vi "Calibration.vi"(4 "flush duration [s]":dbl, 7 "Desired Refresh Ratio":dbl=25.0 format="%#_g %", 8 "LINX Resource":T2={"IO"=enum."Remote", "Interface"=enum."TCP", "LINX Device Config"={"Interface"=enum."Serial", "COM Port"="COM13", "TCP Configuration"={"IP Address"="", "Port"=0}, "Device Family"=1, "Device ID"=1, "Device Name"="myRIO-1900", "TCP Ref"=refnum, "Channels"={"DI"=[0, 1, 2, 3, 4, 5, 6, 7, 8, 9, 10, 11, 12, 13, 14, 15, 16, 17, 18, 19, 20, 21, 22, 23, 24, 25, 26, 27, 28, 29, 30, 31, 32, 33, 34, 35, 36, 37, 38, 39, 40, 41, 42, 43, 44, 45, 46], "DO"=[0, 1, 2, 3, 4, 5, 6, 7, 8, 9, 10, 11, 12, 13, 14, 15, 16, 17, 18, 19, 20, 21, 22, 23, 24, 25, 26, 27, 28, 29, 30, 31, 32, 33, 34, 35, 36, 37, 38, 39, 40, 41, 42, 43, 44, 45, 46], "AI"=[0, 1, 2, 3, 4, 5, 6, 7, 8, 9, 10, 11], "AO"=[], "PWM"=[3, 5, 6, 9, 10], "QE"=[], "UART"=[0, 1], "I2C 2"=[0], "SPI"=[0], "CAN"=[], "Servo"=[], "AI Ref (V)"=0.0, "AI Resolution (Bits)"=0, "AO Ref (V)"=0.0, "AO Resolution (Bits)"=0}}}, 9 "SOLA ID":u32, 10 "TANGO ID":i32, 11 "IX 81 Port":refnum<visa-resource-name>="IX2-UCB") -> (0 "error IO":errorcluster, 2 "CalibFile":path, 3 "Number of pump steps\n for the desired refresh ratio":dbl)   [LabVIEW 2018]
doc: "This template is for the Queued Message Handler design pattern.\n\nThe Event Handling Loop generates messages based on user interface actions.\n\nThe Message Handling Loop processes messages generated by the Event Handling Loop, or by other messages. The messages are string values, so new messages can be added easily to the Message Cases case structure in the Message Handling Loop. Each message cluster can also provide an optional value for Message Data, which is a variant that can be converted to whatever message-specific data is required."
uses:
  ANDOR/OwnVIs/AndorOWN.lvlib
  SOLA/LabVIEW 2015 Library (32bit)/LumencorDLL32/LumencorDLL32.lvlib
  Olympus IX BX Series/Olympus IX BX Series.lvlib
  TANGO Stage/TangoOWN.lvlib
  <vilib>/MakerHub/LINX/LMH-LINX.lvlib
  Arduino/VIs/Arduino.lvlib
  ANDOR/Andor SDK/AndorSDK.lvlib
  <vilib>/vision/NI_Vision_Development_Module.lvlib
  tiff/LVTiffWriter/LVTiffWriter.lvlib
  <vilib>/MakerHub/LINX/Public/Peripherals/Digital/Digital Write N Chans.vi
  Calib/Calibration.lvlib
  <vilib>/MakerHub/LINX/Private/Type Defs/Platform.ctl
  <vilib>/MakerHub/LINX/Private/Type Defs/Interface.ctl
  <vilib>/MakerHub/LINX/Private/Device/Type Defs/TCP Config.ctl
  <vilib>/MakerHub/LINX/Private/Device/Device.lvlib
  <vilib>/MakerHub/LINX/Private/Device/Type Defs/Channels.ctl
  <vilib>/MakerHub/LINX/Private/Device/Type Defs/LINX Device Config.ctl
  <vilib>/MakerHub/LINX/Private/Type Defs/LINX Ref.ctl
  C:/Users/Familie/Documents/LabviewIX81/lib/tiff/LVTiffWriter/BitMiracle.LibTiff.NET.dll
  tiff/LVTiffWriter/BitMiracle.LibTiff.NET.dll
panel:
  out "function return":u32
  out "color":string
  in  "Messages":string
  out "TiffHandle":refnum<k24>
  in  "Image Name":string="TestIMG"
  out "Acq. Error Array":cluster{i32, string}[](array[cluster])
  in  "Single Image":bool
  out "Image":T1(plugin-control)
  in  "Colormap":u16(ring) items=["Grey", "Hot"]
  in  "Format":u16(ring)=6
  in  "Path":path
  in  "Save Image":bool
  in  "Exposure 2":sgl=50.0 format="%#_g ms"
  in  "Filter":u16(ring) items=["UV ", "CFP", "GFP", "YFP", "RFP", "BF (empty)"]
  out "exposure out":sgl
  out "accumulate out":sgl
  out "kinetic out":sgl
  out "Camera Temperature":sgl format="%.2f °C"
  in  "Calibrate at Startup":bool
  out "Y Limits":dbl[](array[numeric]) caption="Y Limits [µm]" format="%#_12f"
  out "X Limits":dbl[](array[numeric]) caption="X Limits [µm]" format="%#_10f"
  out "Lower Limit":dbl
  out "Upper Limit":dbl
  in  "Focus [um]":dbl format="%.3f"
  in  "Intensity [%]":dbl(slide) scale=0.0..100.0 scale format="%.1f"
  in  "Light Source":u16(ring) items=["BF - Lamp", "SOLA"]
  in  "Prism Position (1: Bi)":enum16{"Bi", "Side"}(ring)=enum."Side"
  in  "Objective":enum16{"x 4", "x 10", "x 20", "x 40", "x 100"}(ring)=enum."x 10"
  in  "Lamp Type (0: Transmitted)":enum16{"Transmitted", "Reflected"}(ring)
  in  "Enable Lamp":bool
  in  "Shutter":bool
  in  "Microscope Settings":i32(listbox)
  out "Slide":u8(slide) scale=0.0..100.0
  in  "Valve Actuation":i32(listbox)
  in  "Configuration File Path":path
  in  "stop":bool
  out "error out":errorcluster
  in  "Position List":i32[](listbox)
  out "Tango Success":bool
  in  "TANGO COM Port":refnum<visa-resource-name>="COM4"
  in  "SOLA COM Port":refnum<visa-resource-name>="COM5"
  in  "Valve Port (Arduino)":refnum<visa-resource-name>="COM7"
  # "Initialization"
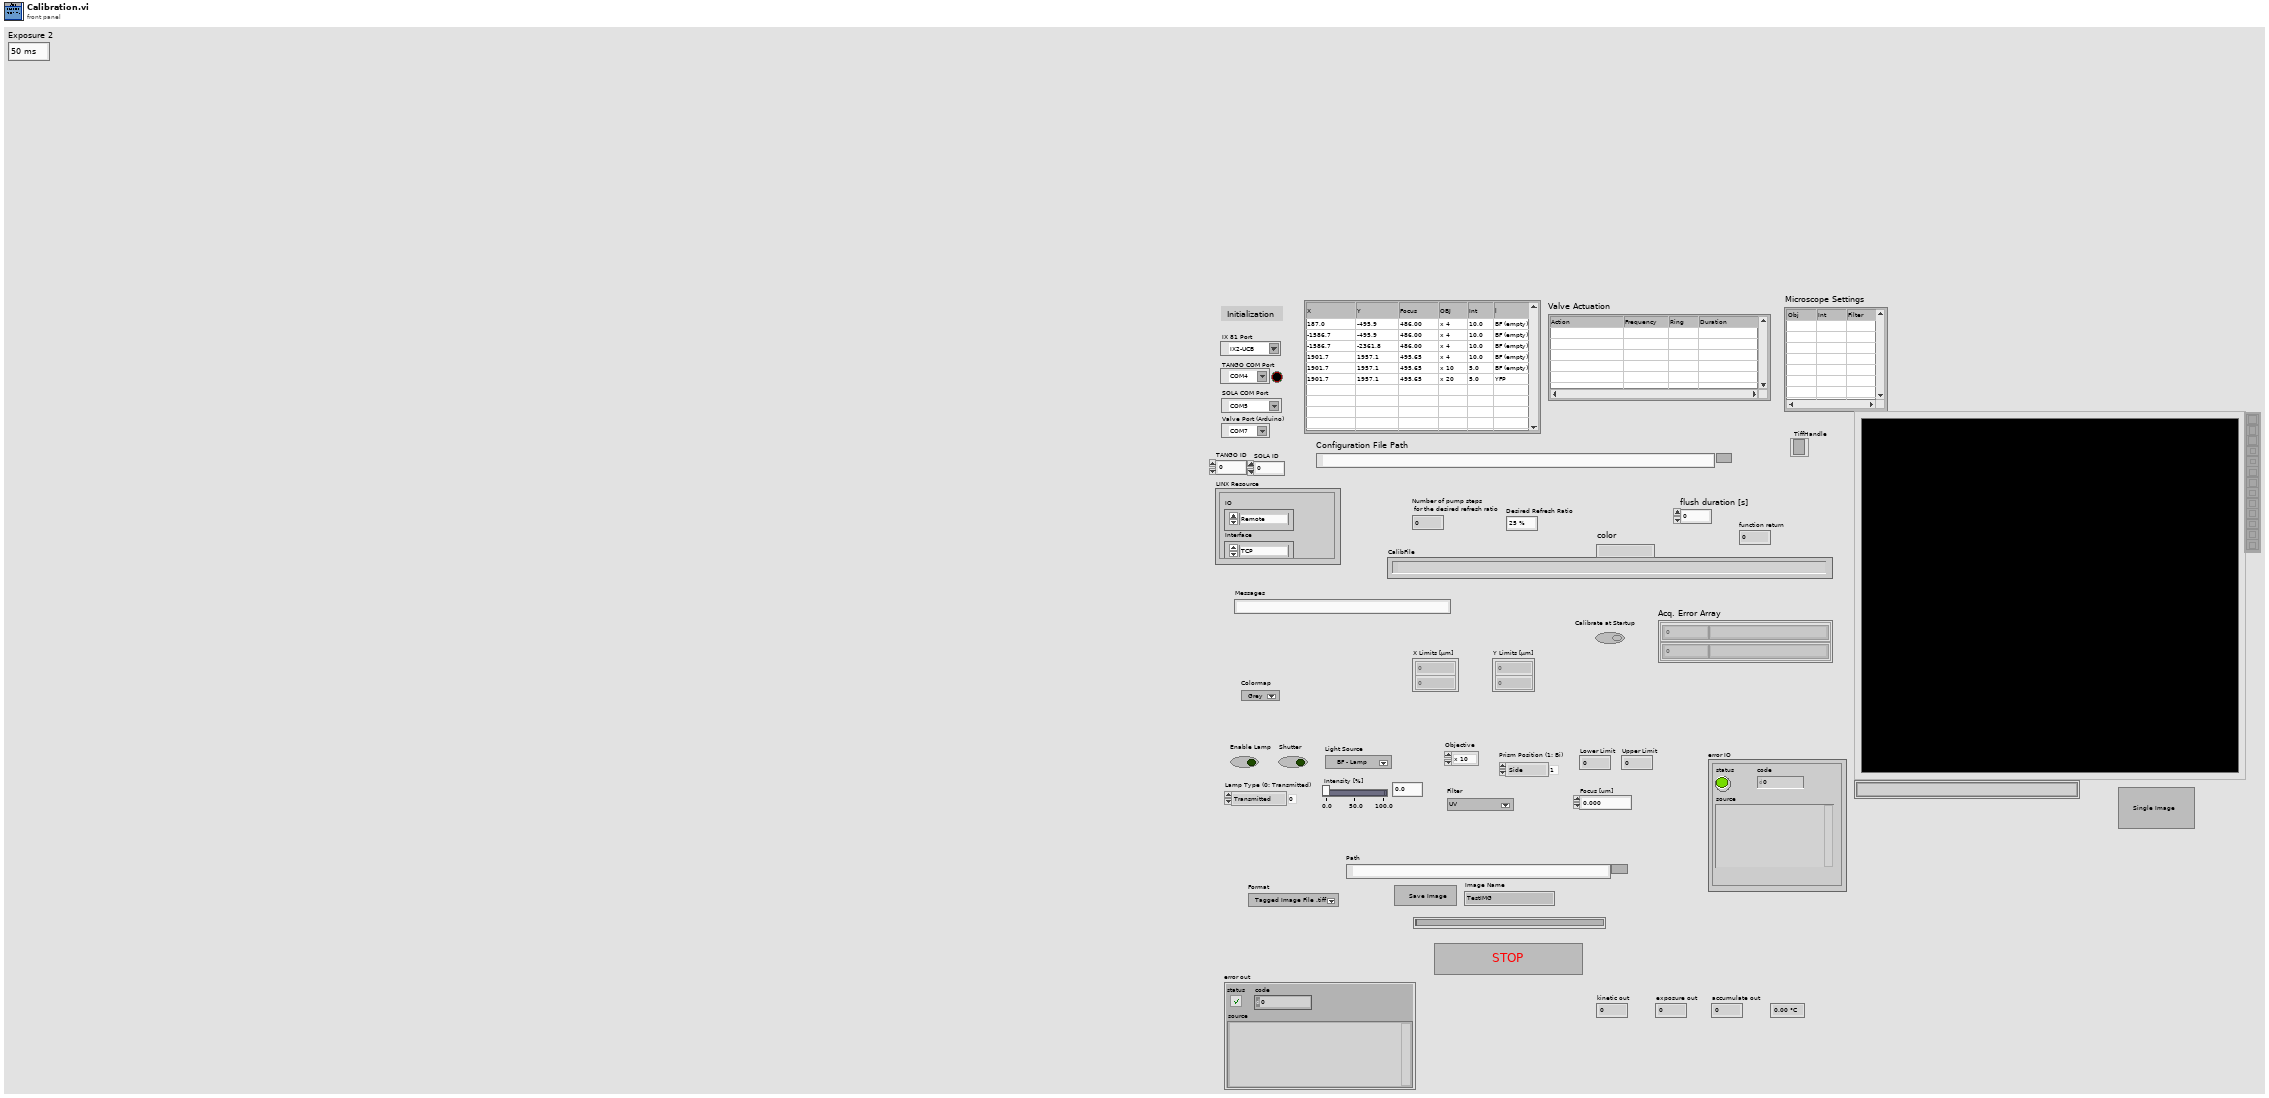
[diagram p1: front panel]
types:
  T1 = typedef "IMAQ Image.ctl" = refnum<image>
  T2 = typedef "LMH-LINX.lvlib/LINX Ref.ctl" = cluster{"IO":T3, "Interface":T4, "LINX Device Config":T5}
  T3 = typedef "LMH-LINX.lvlib/Platform.ctl" = enum16{"Remote", "Local"}
  T4 = typedef "LMH-LINX.lvlib/Interface.ctl" = enum16{"Serial", "TCP"}
  T5 = typedef "LMH-LINX.lvlib/Device.lvlib/LINX Device Config.ctl" = cluster{"Interface":T4, "COM Port":refnum<visa-resource-name>, "TCP Configuration":T6, "Device Family":u8, "Device ID":u8, "Device Name":string, "TCP Ref":refnum<k5>, "Channels":T7}
  T6 = typedef "LMH-LINX.lvlib/Device.lvlib/TCP Config.ctl" = cluster{"IP Address":string, "Port":u16}
  T7 = typedef "LMH-LINX.lvlib/Channels.ctl" = cluster{"DI":u8[], "DO":u8[], "AI":u8[], "AO":u8[], "PWM":u8[], "QE":u8[], "UART":u8[], "I2C 2":u8[], "SPI":u8[], "CAN":u8[], "Servo":u8[], "AI Ref (V)":dbl, "AI Resolution (Bits)":u8, "AO Ref (V)":dbl, "AO Resolution (Bits)":u8}
  T8 = enum16{"open", "replace", "create", "open or create", "replace or create", "replace or create with confirmation"}
  T9 = typedef "Image Type" = u32
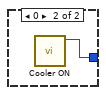
[diagram p2: hidden frame]
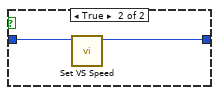
[diagram p3: hidden frame]
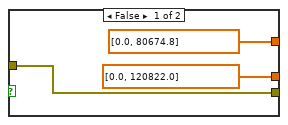
[diagram p4: hidden frame]
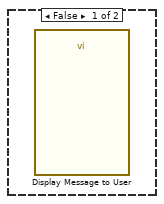
[diagram p6: hidden frame]
diagram:
  n1 = flat-sequence {
    tunnel: [errorcluster {"status"=FALSE, "code"=0, "source"=""} ("error IO")] -> w2
    tunnel: w2 -> [w5]
    tunnel: [w4] -> w1
    tunnel: w1 -> [_]
    frame #0 {
    }
    frame #1 {
      w67 = 0  # openingtime
      w65 = 0  # Auto Mode
      w64 = 1  # TTL High to open
      w66 = 0  # closingtime
      w63 = 0  # Internal Trigger
      w61 = 1  # Single Scan
      w62 = 4  # Image Read
      n2 = call "Is Cooler On.vi"() -> ("function return"=w50:u32, "iCoolerStatus out"=w51:i32)  [unwired: 9 in, 1 out]
      n3 = local read "Calibrate at Startup"() -> (w84:bool)
      n4 = call "lm Color Level.vi"("error in (no error)"=w5, "str_Level"="100", "str_Color"="WHITE") -> ("error out"=w86:errorcluster, "str_Color out"=w87:string)  [unwired: 6 in, 1 out]
      n5 = call "Get VS Speed.vi"() -> ("speed out"=w70:sgl, "function return"=w37:u32)  [unwired: 9 in, 1 out]
      n6 = call "Get Fastest Recommended VS Speed.vi"() -> ("function return"=w36:u32, "speed out"=w69:sgl, "index out"=w72:i32)  [unwired: 8 in, 1 out]
      n7 = case shown="1, Default" w51 {
        tunnel: [u32 20002 ("function return") w91] -> w49
        frame 1, Default {
        }
        frame 0 {
          n8 = call "Cooler ON.vi"() -> ("function return"=w91:u32)  [unwired: 10 in, 1 out]
        }
      }
      n9 = Greater Or Equal?(x=w69, y=w70) -> (x >= y?=w71:bool)
      n10 = call "AndorCreaterErrorCluster.vi"() -> ("Error Code Array"=w35:cluster{i32, string}[])  [unwired: 11 in]
      n11 = call "lm Color Enable.vi"("error in (no error)"=w86, "str_State"="ON", "str_Color"=w87) -> ("error out"=w75:errorcluster)  [unwired: 6 in, 2 out]
      n12 = case shown="True" w84 {
        tunnel: [w95 w102] -> w74
        tunnel: w5 -> [w95 w98]
        tunnel: [dbl[] [0.0, 80674.8] ("Y Limits") w101] -> w82
        tunnel: [dbl[] [0.0, 120822.0] ("X Limits") w100] -> w83
        frame False {
        }
        frame True {
          n13 = local read "TANGO ID"() -> (w99:i32)
          n14 = call "TangoCalibrate.vi"("error in (no error)"=w98, "plLSID in"=w99) -> ("error out"=w102:errorcluster, "X Limits"=w100:dbl[], "Y Limits"=w101:dbl[])  [unwired: 7 in]
        }
      }
      n15 = case shown="False" w71 {
        tunnel: w72 -> [_ w94]
        tunnel: [u32 20002 ("function return") w93] -> w38
        frame False {
        }
        frame True {
          n16 = call "Set VS Speed.vi"("index"=w94) -> ("function return"=w93:u32)  [unwired: 10 in]
        }
      }
      n17 = call "AndorReturn2Error.vi"(9:w35, "Camera return"=w50) -> ("error out"=w33:errorcluster, 3:w34)  [unwired: 8 in]
      n18 = call "AndorReturn2Error.vi"("error in (no error)"=w33, 9:w34, "Camera return"=w49) -> ("error out"=w32:errorcluster, 3:w6)  [unwired: 7 in]
      n19 = call "AndorReturn2Error.vi"("error in (no error)"=w32, 9:w6, "Camera return"=w36) -> ("error out"=w31:errorcluster, 3:w7)  [unwired: 7 in]
      n20 = call "AndorReturn2Error.vi"("error in (no error)"=w31, 9:w7, "Camera return"=w37) -> ("error out"=w30:errorcluster, 3:w8)  [unwired: 7 in]
      n21 = call "AndorReturn2Error.vi"("error in (no error)"=w30, 9:w8, "Camera return"=w38) -> ("error out"=w29:errorcluster, 3:w9)  [unwired: 7 in]
      n22 = call "Get Temperature F.vi"() -> ("function return"=w39:u32, "temperature out"=w68:sgl)  [unwired: 9 in, 1 out]
      n23 = local read "LINX Resource"() -> (w81:T2)
      n24 = local write "Y Limits"(w82) -> ()
      n25 = local write "X Limits"(w83) -> ()
      n26 = local write "Camera Temperature"(w68) -> ()
      n27 = call "AndorReturn2Error.vi"("error in (no error)"=w29, 9:w9, "Camera return"=w39) -> ("error out"=w28:errorcluster, 3:w10)  [unwired: 7 in]
      n28 = call "Set Read Mode.vi"("mode"=w62) -> ("function return"=w40:u32)  [unwired: 9 in, 1 out]
      n29 = call "ArdnoValve2Linx.vi"("error in (no error)"=w5, "Valve (A1-C8),\n comma separated"="A1,A2,A3,A4,A5,A6,A7,A8,B1,B2,B3,B4,B5,B6,B7,B8,C1,C2,C3,C4,C5,C6,C7,C8" ("Valve (A1-C8),\n comma separated")) -> ("error out"=w79:errorcluster, "Closed State"=w78:bool[], "Linx Port"=w77:i32[])  [unwired: 7 in]
      n30 = call "Set Shutter.vi"("openingtime"=w67, "closingtime"=w66, "mode"=w65, "typ"=w64) -> ("function return"=w41:u32)  [unwired: 6 in, 1 out]
      n31 = call "AndorReturn2Error.vi"("error in (no error)"=w28, 9:w10, "Camera return"=w40) -> ("error out"=w27:errorcluster, 3:w11)  [unwired: 7 in]
      n32 = call-poly <vilib>:"Digital Write.vi"("Error In"=w79, "Values"=w78, "DO Channels"=w77, "LINX Resource"=w81) -> ("Error Out"=w76:errorcluster)  [unwired: 6 in, 1 out]
      n33 = call "AndorReturn2Error.vi"("error in (no error)"=w27, 9:w11, "Camera return"=w41) -> ("error out"=w26:errorcluster, 3:w12)  [unwired: 7 in]
      n34 = call "Set Trigger Mode.vi"("mode"=w63) -> ("function return"=w42:u32)  [unwired: 9 in, 1 out]
      n35 = call "Set Acquisition Mode.vi"("mode"=w61) -> ("function return"=w43:u32)  [unwired: 9 in, 1 out]
      n36 = call "AndorReturn2Error.vi"("error in (no error)"=w26, 9:w12, "Camera return"=w42) -> ("error out"=w25:errorcluster, 3:w13)  [unwired: 7 in]
      n37 = call "AndorReturn2Error.vi"("error in (no error)"=w25, 9:w13, "Camera return"=w43) -> ("error out"=w24:errorcluster, 3:w14)  [unwired: 7 in]
      n38 = call "Set Temperature.vi"("temperature"=-60) -> ()  [unwired: 9 in, 2 out]
      n39 = call "Set Frame Transfer Mode.vi"("mode"=1) -> ("function return"=w44:u32)  [unwired: 10 in]
      n40 = call "AndorReturn2Error.vi"("error in (no error)"=w24, 9:w14, "Camera return"=w44) -> ("error out"=w23:errorcluster, 3:w15)  [unwired: 7 in]
      n41 = local read item#-1() -> (w57)
      n42 = call "Set Number Accumulations.vi"("number"=1) -> ("function return"=w45:u32)  [unwired: 9 in, 1 out]
      n43 = call "AndorReturn2Error.vi"("error in (no error)"=w23, 9:w15, "Camera return"=w45) -> ("error out"=w22:errorcluster, 3:w16)  [unwired: 7 in]
      n44 = Divide(x=w57, y=sgl 1000.0) -> (x/y=w56:sgl)
      n45 = call "Set Number Kinetics.vi"("number"=1) -> ("function return"=w46:u32)  [unwired: 9 in, 1 out]
      n46 = call "Set Exposure Time.vi"("time"=w56) -> ("function return"=w47:u32)  [unwired: 9 in, 1 out]
      n47 = call "AndorReturn2Error.vi"("error in (no error)"=w22, 9:w16, "Camera return"=w46) -> ("error out"=w21:errorcluster, 3:w17)  [unwired: 7 in]
      n48 = call "AndorReturn2Error.vi"("error in (no error)"=w21, 9:w17, "Camera return"=w47) -> ("error out"=w20:errorcluster, 3:w18)  [unwired: 7 in]
      n49 = call "Get Acquisition Timings.vi"() -> ("kinetic out"=w54:sgl, "accumulate out"=w52:sgl, "exposure out"=w53:sgl, "function return"=w48:u32)  [unwired: 7 in, 1 out]
      n50 = call "AndorReturn2Error.vi"("error in (no error)"=w20, 9:w18, "Camera return"=w48) -> ("error out"=w19:errorcluster)  [unwired: 8 in]
      n51 = local write "exposure out"(w53) -> ()
      n52 = local write "accumulate out"(w52) -> ()
      n53 = local write "kinetic out"(w54) -> ()
      n54 = Merge Errors(w76, w75, w74, w19) -> (w4:errorcluster)
    }
    frame #2 {
      n55 = Two Button Dialog(message="Do you want to calibrate the pumps now?") -> (T button?=w103:bool)  [unwired: 2 in]
      n56 = case shown="True" w103 {
        frame False {
        }
        frame True {
          n57 = flat-sequence {
            tunnel: [w149] -> w107
            tunnel: w107 -> [w153]
            tunnel: [w153] -> w106
            tunnel: [w151] -> w105
            tunnel: w106 -> [w155]
            tunnel: w105 -> [w154]
            frame #0 {
              n58 = Open/Create/Replace File(prompt="Specify the .tif file to save the images in.", operation (0:open)=T8."create", access (0:read/write)=enum16{"read/write", "read-only", "write-only"}."read/write") -> (refnum out=w111:refnum<file>, error out=w112:errorcluster)  [unwired: 3 in, 1 out]
              n59 = Close File(refnum=w111, error in=w112) -> (path=w110:path)  [unwired: 1 out]
              "CalibFile" <- w110
              n60 = call "tiffOpenForWrite.vi"("Path"=w110) -> ("TiffOut"=→"TiffHandle":refnum<k24>)  [unwired: 10 in]
            }
            frame #1 {
              w121 = u16 1 items=["BF - Lamp", "SOLA"] ("Light Source")
              n61 = call "Exposure Time check"() -> ("Color"=w115:string, "Exposure Time  [ms]"=w116:dbl)  [unwired: 16 in, 2 out]
              "color" <- w115
              n62 = local write "Light Source"(w121) -> ()
              n63 = property on="Filter" class="Ring (strict)"() -> ("Strings []"=w120:string[])  [unwired: 2 in, 2 out]
              n64 = Array Size(array=w120) -> (size(s)=w118:i32)
              n65 = flat-sequence {
                tunnel: [w134] -> w122
                tunnel: w116 -> [w135]
                tunnel: w122 -> [w145]
                frame #0 {
                  n66 = while {
                    tunnel: w135 -> [w136]
                    tunnel: [w136] -> w134
                    stop <- w137 stop-if-true
                    n67 = call "Get Status.vi"() -> ("function return"=w143:u32, "status out"=w140:i32)  [unwired: 9 in, 1 out]
                    n68 = Equal?(x=20073 ("status out"), y=w140) -> (x = y?=w139:bool)
                    n69 = Equal?(x=w143, y=20002 ("x")) -> (x = y?=w138:bool)
                    n70 = And(x=w139, y=w138) -> (x .and. y?=w137:bool)
                  }
                }
                frame #1 {
                  n71 = Divide(x=w145, y=sgl 1000.0) -> (x/y=w147:dbl)
                  n72 = call "Set Exposure Time.vi"("time"=w147) -> ("function return"=→"function return":u32)  [unwired: 9 in, 1 out]
                }
              }
              n73 = for {
                N: w118 -> [_]
                tunnel: w120 -> [w132] mode=indexing
                tunnel: w115 -> [w131]
                tunnel: [w130] -> w117
                i -> [w130]
                stop <- w133 stop-if-true
                n74 = Equal?(x=w131, y=w132) -> (x = y?=w133:bool)
              }
              n75 = local write item#-1(w116) -> ()
              n76 = Less?(x=w117, y=w118) -> (x < y?=w119:bool)
              n77 = case shown="True" w119 {
                tunnel: w117 -> [_ w126]
                frame False {
                  n78 = call "Display Message to User"() -> ()  [unwired: 10 in, 2 out]
                }
                frame True {
                  n79 = Increment(x=w126) -> (x+1=w125:i32)
                  n80 = Number To Decimal String(number=w125) -> (decimal integer string=w127:string)  [unwired: 1 in]
                  n81 = call <vilib>:"Space Constant.vi"() -> ("String"=w129:string)
                  n82 = local read "IX 81 Port"() -> (w123:refnum<visa-resource-name>)
                  n83 = Concatenate Strings("MU", w129, w127) -> (w124:string)
                  n84 = call "OlympusQuery.vi"("String"=w124, "VISA Resource Name In"=w123) -> ()  [unwired: 7 in, 3 out]
                }
              }
            }
            frame #2 {
            }
            frame #3 {
              n85 = local read "LINX Resource"() -> (w150:T2)
              n86 = One Button Dialog(message="Please load the fluorophore now") -> ()  [unwired: 1 in, 1 out]
              n87 = call "AndorConvertErrCodeToMessage.vi"(11:w150) -> (3:w149)  [unwired: 9 in, 1 out]
            }
            frame #4 {
              n88 = One Button Dialog(message="Please load the dilutant now") -> (true=w151:bool)  [unwired: 1 in]
            }
            frame #5 {
              n89 = case shown="True" w154 {
                tunnel: w155 -> [_ w156]
                frame False {
                }
                frame True {
                  n90 = flat-sequence {
                    tunnel: [w161] -> w159
                    tunnel: w156 -> [w160]
                    tunnel: w159 -> [w166]
                    tunnel: [w166] -> w158
                    tunnel: w158 -> [w169]
                    tunnel: [w167] -> w157
                    frame #0 {
                      n91 = call "ArdnoFlush.vi"("Open?"=FALSE, "Single / Multivalve?"=FALSE, "Channel"=u32 1, "LINX Resource"=w160) -> ("LINX Resource out"=w161:T2)  [unwired: 6 in, 1 out]
                    }
                    frame #1 {
                      n92 = Wait (ms)(milliseconds to wait="flush duration [s]") -> ()  [unwired: 1 out]
                    }
                    frame #2 {
                      (unwired) u32 1 ("Channel")
                      n93 = call "ArdnoFlush.vi"("Open?"=TRUE, "Single / Multivalve?"=FALSE, "LINX Resource"=w169) -> ("LINX Resource out"=w167:T2)  [unwired: 7 in, 1 out]
                    }
                  }
                  n94 = while {
                    tunnel: w157 -> [w178]
                    i -> [w175]
                    stop <- w172 continue-if-true
                    n95 = flat-sequence {
                      tunnel: w178 -> [w186]
                      tunnel: [w182] -> w177
                      tunnel: [w181] -> w176
                      tunnel: w177 -> [w191]
                      tunnel: w176 -> [w190]
                      tunnel: w175 -> [w192]
                      frame #0 {
                        w180 = u32 8  # Frequency
                        w184 = 15  # Feed Cycles
                        w185 = u32 1  # Channel
                        n96 = call "ArdnoFeed.vi"("LINX Resource"=w186, "Single / Multiring?"=FALSE ("Single / Multivalve?"), "Channel"=w185, "Feed Cycles"=w184, 13:w180) -> ("LINX Resource out"=w182:T2, "error out"=w181:errorcluster)  [unwired: 8 in, 1 out]
                      }
                      frame #1 {
                        w187 = 10  # Pump Frequency
                        w189 = 4  # Pump Cycles
                        n97 = call "ArdnoPump.vi"("LINX Resource"=w191, "Pump Cycles"=w189, "Pump Frequency"=w187, "error in (no error)"=w190, "Single/\nMultiring?"=FALSE ("Single/\nMultiring?")) -> ()  [unwired: 2 out]
                      }
                      frame #2 {
                        n98 = flat-sequence {
                          tunnel: TRUE ("NewVal") -> [w201]
                          tunnel: [w201] -> w196
                          tunnel: [w205] -> w195
                          tunnel: w196 -> [w205]
                          tunnel: w193 -> [w207]
                          tunnel: w195 -> [w208]
                          tunnel: w192 -> [w206]
                          frame #0 {
                            w199 = 1  # Single Scan
                            w200 = 4  # Image Read
                            n99 = call "Set Number Accumulations.vi"("number"=1) -> ()  [unwired: 9 in, 2 out]
                            n100 = call "Set Acquisition Mode.vi"("mode"=w199) -> ()  [unwired: 9 in, 2 out]
                            n101 = call "Set Read Mode.vi"("mode"=w200) -> ()  [unwired: 9 in, 2 out]
                            n102 = call "Set Number Kinetics.vi"("number"=1) -> ()  [unwired: 9 in, 2 out]
                          }
                          frame #1 {
                            n103 = local read item#-1() -> (w202)
                            n104 = Divide(x=w202, y=sgl 1000.0) -> (x/y=w204:sgl)
                            n105 = call "Set Exposure Time.vi"("time"=w204) -> ()  [unwired: 9 in, 2 out]
                          }
                          frame #2 {
                            n106 = case shown="True" w208 {
                              tunnel: w207 -> [_ w219]
                              tunnel: w206 -> [_ w209]
                              frame False {
                              }
                              frame True {
                                n107 = flat-sequence {
                                tunnel: w219 -> [w220]
                                tunnel: [w222] -> w218
                                tunnel: [w221] -> w217
                                tunnel: w218 -> [w224]
                                tunnel: w217 -> [w225]
                                tunnel: [w225] -> w216
                                tunnel: [w224] -> w215
                                tunnel: w216 -> [w240]
                                tunnel: w215 -> [w239]
                                tunnel: [w240] -> w214
                                tunnel: [w239] -> w213
                                tunnel: [w235] -> w212
                                tunnel: [w236] -> w211
                                tunnel: w214 -> [w244]
                                tunnel: w213 -> [w242]
                                tunnel: w212 -> [w243]
                                tunnel: w211 -> [w246]
                                tunnel: [w246] -> w210
                                tunnel: w210 -> [w269]
                                tunnel: w209 -> [w249]
                                frame #0 {
                                n108 = call "Start Acquisition.vi"() -> ("function return"=w223:u32)  [unwired: 10 in, 1 out]
                                n109 = call "Calibration.vi"("LINX Resource"=w223, "IX 81 Port"=w220) -> ("error IO"=w221:errorcluster, "Number of pump steps\n for the desired refresh ratio"=w222:dbl)  [unwired: 7 in, 1 out]
                                }
                                frame #1 {
                                n110 = while {
                                stop <- w226 stop-if-true
                                n111 = call "Get Status.vi"() -> ("function return"=w232:u32, "status out"=w229:i32)  [unwired: 9 in, 1 out]
                                n112 = Equal?(x=20073 ("status out"), y=w229) -> (x = y?=w228:bool)
                                n113 = Equal?(x=w232, y=20002 ("x")) -> (x = y?=w227:bool)
                                n114 = And(x=w228, y=w227) -> (x .and. y?=w226:bool)
                                }
                                }
                                frame #2 {
                                n115 = Square(x=1024) -> (x^2=w233:i32)
                                n116 = Initialize Array(i16 0 ("element"), w233) -> (w234:i16[])
                                n117 = call "Get Most Recent Image16.vi"("size"=w233, "arr"=w234) -> ("function return"=w235:u32, "arr out"=w236:i16[])  [unwired: 7 in, 1 out]
                                }
                                frame #3 {
                                n118 = call "Calibration.vi"("LINX Resource"=w243, "IX 81 Port"=w242) -> ("error IO"=w245:errorcluster)  [unwired: 7 in, 2 out]
                                n119 = Build Array(w245, w244) -> (w241:errorcluster[])
                                n120 = local write "Acq. Error Array"(w241) -> ()
                                }
                                frame #4 {
                                w272 = u32 2 items=["Zero Order", "Bi-Linear", "Quadratic", "Cubic Spline"] ("Interpolation Type")
                                w271 = T9 7 items=["Grayscale (U8)", "Grayscale (I16)", "Grayscale (SGL)", "Complex (CSG)", "RGB (U32)", "HSL (U32)", "RGB (U64)", "Grayscale (U16)"] ("Image Type")
                                w270 = 1024 ("dimension size")
                                n121 = Add(x=1 ("y"), y=w249) -> (x+y=w254:i32)
                                n122 = local read "Image Name"() -> (w268:string)
                                n123 = Reshape Array(w269, w270, w270) -> (w248:i16[][])
                                n124 = To Unsigned Word Integer(number=w248) -> (unsigned 16bit integer=w247:u16[][])
                                n125 = call "IMAQ Create"("Image Name"=w268, "Image Type"=w271) -> ("New Image"=w273:T1)  [unwired: 3 in, 1 out]
                                n126 = Bundle By Name(cluster=cluster{"Page":i32, "TotalPages":i32} {"Page"=0, "TotalPages"=0} ("Multipage"), "TotalPages"=10, "Page"=w254) -> (w256:cluster{"Page":i32, "TotalPages":i32})
                                n127 = local read "TiffHandle"() -> (w258:refnum<k24>)
                                n128 = call "IMAQ ArrayToImage"("Image Pixels (U16)"=w247, "Image"=w273) -> ("Image Out"=w253:T1)  [unwired: 8 in, 1 out]
                                n129 = property on="Image" class="ImageControl"() -> ("Image Area Height"=w266:u32, "Image Area Width"=w267:u32)  [unwired: 2 in, 2 out]
                                n130 = call "tiffWriteImaqToTiff.vi"("Multipage"=w256, "ImaqIn"=w253, "TiffIn"=w258) -> ("ImaqOut"=w252:T1, "TiffOut"=w259:refnum<k24>)  [unwired: 7 in]
                                n131 = call "IMAQ GetImageSize"("Image"=w253) -> ("Y Resolution"=w260:i32, "X Resolution"=w263:i32)  [unwired: 3 in, 1 out]
                                n132 = Divide(x=w260, y=w266) -> (x/y=w274:dbl)
                                n133 = Divide(x=w263, y=w267) -> (x/y=w275:dbl)
                                n134 = local write "TiffHandle"(w259) -> ()
                                n135 = Max & Min(x=w274, y=w275) -> (max(x,y)=w265:dbl, min(x,y)=w261:dbl)
                                n136 = Divide(x=w263, y=w265) -> (x/y=w264:dbl)
                                n137 = Divide(x=w260, y=w261) -> (x/y=w262:dbl)
                                n138 = call "IMAQ Resample"("X Resolution"=w264, "Y Resolution"=w262, "Interpolation Type"=w272, "Image Src"=w252) -> ("Image Dst Out"=w251:T1)  [unwired: 6 in, 1 out]
                                n139 = local write "Image"(w251) -> ()
                                }
                                }
                              }
                            }
                          }
                        }
                        n140 = call "AndorCreaterErrorCluster.vi"() -> ("Error Code Array"=w193:cluster{i32, string}[])  [unwired: 11 in]
                      }
                    }
                    n141 = Not(x="stop") -> (.not. x?=w173:bool)
                    n142 = Less?(x=w175, y=10.0) -> (x < y?=w174:bool)
                    n143 = And(x=w174, y=w173) -> (x .and. y?=w172:bool)
                  }
                }
              }
            }
            frame #6 {
              n144 = local read "stop"() -> (w279:bool)
              n145 = case shown="False" w279 {
                tunnel: [w282 w286] -> w280
                tunnel: errorcluster {"status"=FALSE, "code"=0, "source"=""} ("error constant") -> [w282 w285]
                tunnel: [inf w284] -> w277
                tunnel: "Desired Refresh Ratio" -> [_ w283]
                frame True {
                }
                frame False {
                  n146 = call "CalibComputeRatio.vi"("error in (no error)"=w285, "Desired Refresh Ratio"=w283) -> ("error out"=w286:errorcluster, "Pump steps for the\n desired refresh ratio"=w284:dbl)  [unwired: 8 in]
                }
              }
              "error IO" <- w280
              "Number of pump steps\n for the desired refresh ratio" <- w277
            }
            frame #7 {
            }
          }
        }
      }
    }
  }
